vi "Compare.vi"(10 "Numeric 2":i32, 11 "Numeric 1":i32) -> (3 "Result":T1)   [LabVIEW 2013]
uses:
  Metadata/Compare Results.ctl
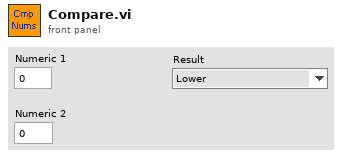
[diagram p1: front panel]
types:
  T1 = typedef "Compare Results.ctl" = enum16{"Lower", "Same", "Higher"}
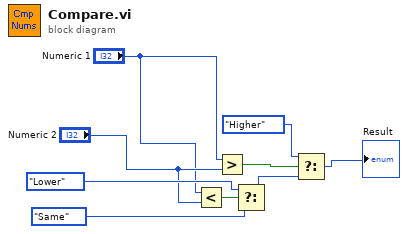
[diagram p0: block diagram]
diagram:
  n1 = Less?(x="Numeric 1", y="Numeric 2") -> (x < y?=w5:bool)
  n2 = Greater?(x="Numeric 1", y="Numeric 2") -> (0:w1:bool)
  n3 = Select(t=Compare_Results."Lower" ("Compare Results"), s=w5, f=Compare_Results."Same") -> (s? t:f=w7:T1)
  n4 = Select(t=Compare_Results."Higher" ("Compare Results"), s=w1, f=w7) -> (s? t:f=→"Result":T1)
